vi "SS2 Live_Abort Saving Tasks.vi"(8 "Error In":errorcluster) -> (0 "Error Out":errorcluster, 2 "Notebook Message":string, 3 "UI Message":string)   [LabVIEW 2019]
uses:
  SS2 Live_Internal Data List.ctl
  SS2 Live_File Saving Task Information.ctl
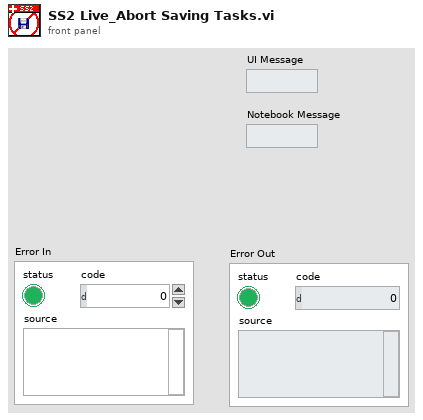
[diagram p1: front panel]
types:
  T1 = typedef "SS2 Live_File Saving Task Information.ctl" = cluster{"File Path":string, "# Saved Images":i32, "# Images (Total)":i32, "File Size (Bytes)":i64}
  T2 = typedef "SS2 Live_Internal Data List.ctl" = enum16{"Number of pending file saving tasks", "File Saving Tasks Information", "Current Image ROI Information", "# FPGA Reset Attempts"}
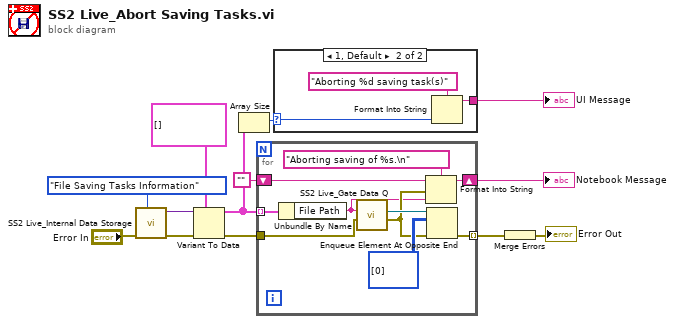
[diagram p0: block diagram]
diagram:
  n1 = call "SS2 Live_Internal Data Storage.vi"("SS2 Live Data"=SS2_Live_Internal_Data_List."File Saving Tasks Information", "Error In"="Error In") -> ("Error Out"=w11:errorcluster, "Variant"=w12:variant)  [unwired: 7 in, 1 out]
  n2 = Variant To Data(error in=w11, type=T1[] [] ("Array"), Variant=w12) -> (data=w3:T1[], error out=w8:errorcluster)
  n3 = Array Size(array=w3) -> (size(s)=w2:i32)
  n4 = for {
    tunnel: w3 -> [w23] mode=indexing
    tunnel: w8 -> [w22]
    tunnel: [w19] -> w7 mode=indexing
    shift-right: [w17] -> w4
    shift-left: "" -> [w18]
    n5 = Unbundle By Name(w23) -> ("File Path"=w15:string)
    n6 = call "SS2 Live_Gate Data Q.vi"("error in (no error)"=w22, "SS2 Live Gate Data Q Name"=w15) -> ("error out"=w16:errorcluster, "SS2 Live Gate Data Q"=w21:refnum<queue>)  [unwired: 4 in]
    n7 = Format Into String(format string="Aborting saving of %s.\n", initial string=w18, error in=w16, w15) -> (resulting string=w17:string)  [unwired: 1 out]
    n8 = Enqueue Element At Opposite End(queue=w21, element=u8[][] [[0]], error in (no error)=w16) -> (error out=w19:errorcluster)  [unwired: 1 in, 2 out]
  }
  "Notebook Message" <- w4
  n9 = case shown="1, Default" w2 {
    selector: w2 -> [_ w24]
    tunnel: [_ w26] -> w1
    frame 0 {
    }
    frame 1, Default {
      n10 = Format Into String(format string="Aborting %d saving task(s)" ("UI Message"), w24) -> (resulting string=w26:string)  [unwired: 2 in, 1 out]
    }
  }
  "UI Message" <- w1
  n11 = Merge Errors(w7) -> (→"Error Out":errorcluster)
